vi "PLL -- data source -- V3 -- wrapper.vi"(6 "set-get delay (msec)":i64, 7 "data source action":T2=enum."get", 9 "z  in (V)":cdb, 10 "Freq in (Hz)":dbl=40000.0 format="%#_13g", 11 "PLL data source":T1=enum."MFLI") -> (1 "z out (V)":cdb=0.00010527635459-2.9308681405e-05i, 2 "Freq out (Hz)":dbl=55115.2, 3 "PLL data source OUT":T1=enum."MFLI")   [LabVIEW 2018]
uses:
  PLL data source.ctl
  data source action.ctl
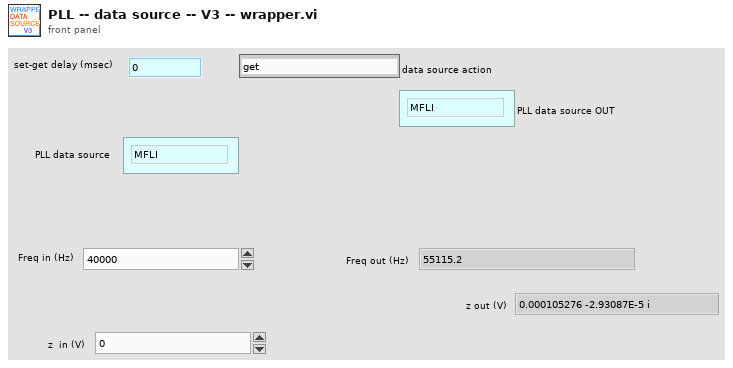
[diagram p1: front panel]
types:
  T1 = typedef "PLL data source.ctl" = enum16{"meta", "MFLI", "SRS865A", "arydh"}
  T2 = typedef "data source action.ctl" = enum16{"set", "get", "init", "set-and-get", "init source"}
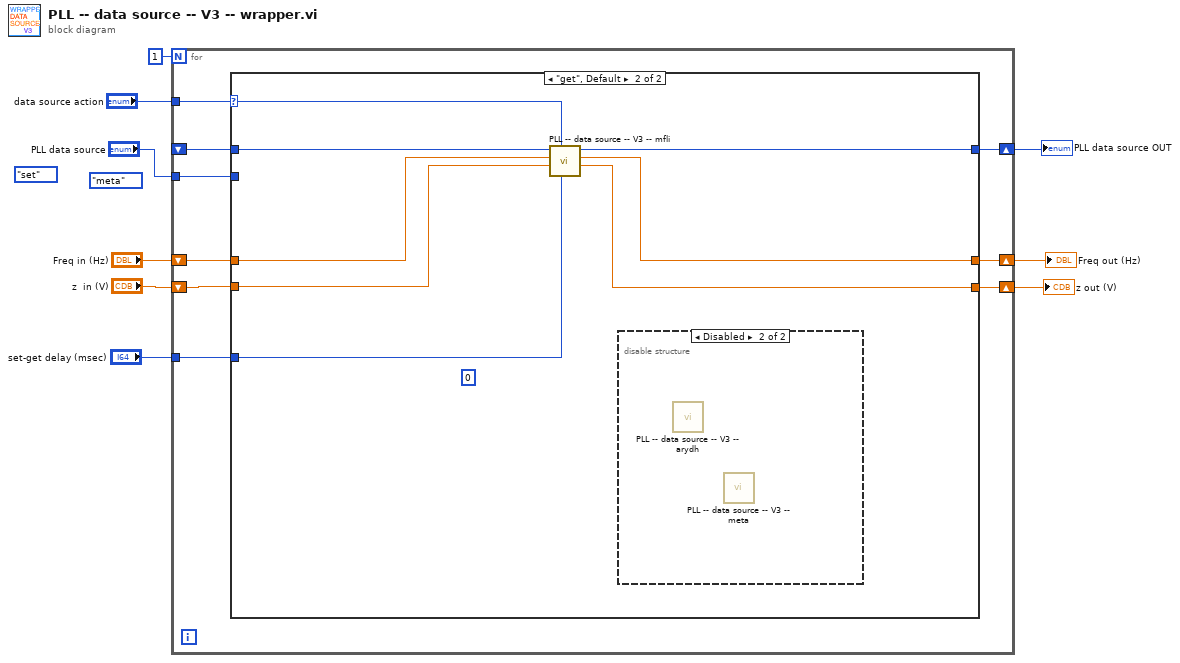
[diagram p0: block diagram]
diagram:
  (unwired) data_source_action."set" ("data source action")
  (unwired) PLL_data_source."meta" ("PLL data source")
  n1 = for {
    N: 1 -> [_]
    tunnel: "data source action" -> [w11]
    tunnel: "set-get delay (msec)" -> [w14]
    shift-right: [w15] -> w6
    shift-left: _ -> [w18]
    shift-right: [w17] -> w8
    shift-left: "Freq in (Hz)" -> [w16]
    shift-right: [w12] -> w3
    shift-left: "z  in (V)" -> [w13]
    tunnel: "PLL data source" -> [w10]
    n2 = case shown="\"get\", Default" w11 {
      selector: w11 -> [_ w27]
      tunnel: w18 -> [_ w29]
      tunnel: [w21 w23] -> w17
      tunnel: w16 -> [w21 w26]
      tunnel: [w19 w28] -> w15
      tunnel: w14 -> [_ w22]
      tunnel: w13 -> [w20 w25]
      tunnel: [w20 w24] -> w12
      tunnel: w10 -> [w19 _]
      frame "init source" {
      }
      frame "get", Default {
        (unwired) i64 0 ("set-get delay (msec)")
        n3 = call "PLL -- data source -- V3 -- mfli.vi"("set-get delay (msec)"=w22, "data source action"=w27, "z  in (V)"=w25, "Freq in (Hz)"=w26, "PLL data source"=w29) -> ("z out (V)"=w24:cdb, "Freq out (Hz)"=w23:dbl, "PLL data source OUT"=w28:T1)  [unwired: 4 in]
        n4 = disable-structure shown="Disabled" {
          frame Enabled {
          }
          frame Disabled {
            n5 = call "PLL -- data source -- V3 -- arydh.vi"() -> ()  [unwired: 9 in, 3 out]
            n6 = call "PLL -- data source -- V3 -- meta.vi"() -> ()  [unwired: 9 in, 3 out]
          }
        }
      }
    }
  }
  "Freq out (Hz)" <- w8
  "z out (V)" <- w3
  "PLL data source OUT" <- w6
